vi "Read Analog Parameters.vi"(8 "error in (no error)":errorcluster, 11 "VISA resource name":refnum<visa-resource-name>) -> (0 "error out":errorcluster, 2 "analog parameters":T1={"aout bounds"={"ABndUpC"=0.0, "ABndUpL"=0.0, "ABndLoC"=0.0, "ABndLoL"=0.0}, "aout cfactor"={"CFactorC"=0.0, "CFactorL"=0.0}, "aout span"={"ASpanC"=20.0, "ASpanL"=20.0}, "aout point"={"APointC"=20.0, "APointL"=20.0}}, 3 "VISA resource name out":refnum<visa-resource-name>)   [LabVIEW 2019, in "Andeen-Hagerling 2700A.lvlib"]
doc: "Read the analog out parameters which may vary with other analog out or deviation paramters. Includes aout bounds, aout span, aout cfactor and aout point."
uses:
  Andeen-Hagerling 2700A.lvlib
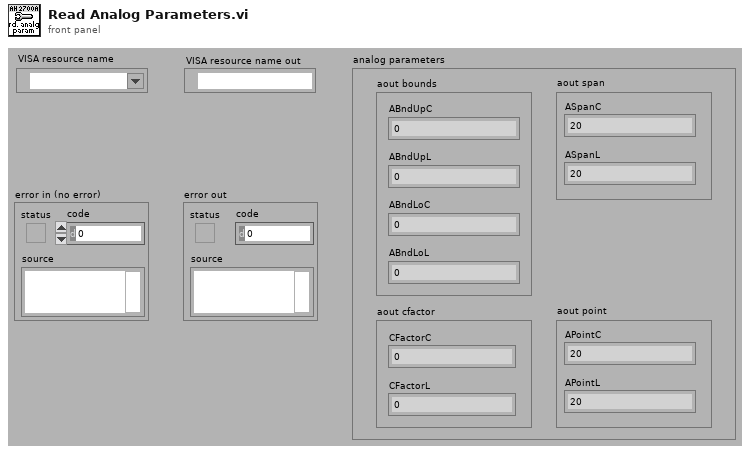
[diagram p1: front panel]
types:
  T1 = cluster{"aout bounds":cluster{"ABndUpC":dbl, "ABndUpL":dbl, "ABndLoC":dbl, "ABndLoL":dbl}, "aout cfactor":cluster{"CFactorC":dbl, "CFactorL":dbl}, "aout span":cluster{"ASpanC":dbl, "ASpanL":dbl}, "aout point":cluster{"APointC":dbl, "APointL":dbl}}
  T2 = cluster{"ABndUpC":dbl, "ABndUpL":dbl, "ABndLoC":dbl, "ABndLoL":dbl}
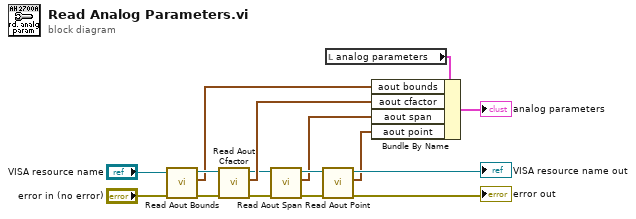
[diagram p0: block diagram]
diagram:
  n1 = call "Read Aout Bounds.vi"("error in (no error)"="error in (no error)", "VISA resource name"="VISA resource name") -> ("error out"=w16:errorcluster, "aout bounds"=w6:T2, "VISA resource name out"=w15:refnum<visa-resource-name>)  [unwired: 7 in]
  n2 = call "Read Aout Cfactor.vi"("error in (no error)"=w16, "VISA resource name"=w15) -> ("error out"=w3:errorcluster, "aout cfactor"=w5:cluster{"CFactorC":dbl, "CFactorL":dbl}, "VISA resource name out"=w4:refnum<visa-resource-name>)  [unwired: 7 in]
  n3 = call "Read Aout Span.vi"("error in (no error)"=w3, "VISA resource name"=w4) -> ("error out"=w13:errorcluster, "aout span"=w2:cluster{"ASpanC":dbl, "ASpanL":dbl}, "VISA resource name out"=w14:refnum<visa-resource-name>)  [unwired: 7 in]
  n4 = call "Read Aout Point.vi"("error in (no error)"=w13, "VISA resource name"=w14) -> ("error out"=→"error out":errorcluster, "aout point"=w1:cluster{"APointC":dbl, "APointL":dbl}, "VISA resource name out"=→"VISA resource name out":refnum<visa-resource-name>)  [unwired: 7 in]
  n5 = local read "analog parameters"() -> (w10:T1)
  n6 = Bundle By Name(cluster=w10, "aout bounds"=w6, "aout cfactor"=w5, "aout span"=w2, "aout point"=w1) -> (→"analog parameters":T1)
